vi "edit_waveform.vi"(8 "error in":errorcluster, 9 "units/sec (ms=1000)":dbl=1000.0, 10 "Clock Rate":dbl=1000000.0 min=0.0, 11 "Channels Control":string[][](table)=[["Hex 3D MOT b0", "1", "0", "", "", "", "", "", "", "", "", "", "", "", "", "", "", "", "", ""], ["Hex 3D MOT b0", "1", "0", "", "", "", "", "", "", "", "", "", "", "", "", "", "", "", "", ""], ["repumper bit0", "1", "0", "", "", "", "", "", "", "", "", "", "", "", "", "", "", "", "", ""], ["Trap Array beam switch", "1", "0", "", "", "", "", "", "", "", "", "", "", "", "", "", "", "", "", ""], ["2D MOT switch", "1", "0", "", "", "", "", "", "", "", "", "", "", "", "", "", "", "", "", ""], ["Hamamatsu CCD trigger", "1", "0", "", "", "", "", "", "", "", "", "", "", "", "", "", "", "", "", ""], ["Luca CCD trigger", "1", "0", "", "", "", "", "", "", "", "", "", "", "", "", "", "", "", "", ""], ["broken", "", "", "", "", "", "", "", "", "", "", "", "", "", "", "", "", "", "", ""], ["repumper bit1", "1", "0", "", "", "", "", "", "", "", "", "", "", "", "", "", "", "", "", ""], ["blow away", "1", "0", "", "", "", "", "", "", "", "", "", "", "", "", "", "", "", "", ""], ["trap shutter", "1", "0", "", "", "", "", "", "", "", "", "", "", "", "", "", "", "", "", ""], ["1038 switch", "1", "0", "", "", "", "", "", "", "", "", "", "", "", "", "", "", "", "", ""], ["", "", "", "", "", "", "", "", "", "", "", "", "", "", "", "", "", "", "", ""], ["", "", "", "", "", "", "", "", "", "", "", "", "", "", "", "", "", "", "", ""], ["", "", "", "", "", "", "", "", "", "", "", "", "", "", "", "", "", "", "", ""], ["", "", "", "", "", "", "", "", "", "", "", "", "", "", "", "", "", "", "", ""], ["", "", "", "", "", "", "", "", "", "", "", "", "", "", "", "", "", "", "", ""], ["", "", "", "", "", "", "", "", "", "", "", "", "", "", "", "", "", "", "", ""], ["", "", "", "", "", "", "", "", "", "", "", "", "", "", "", "", "", "", "", ""], ["", "", "", "", "", "", "", "", "", "", "", "", "", "", "", "", "", "", "", ""], ["", "", "", "", "", "", "", "", "", "", "", "", "", "", "", "", "", "", "", ""], ["", "", "", "", "", "", "", "", "", "", "", "", "", "", "", "", "", "", "", ""], ["", "", "", "", "", "", "", "", "", "", "", "", "", "", "", "", "", "", "", ""], ["", "", "", "", "", "", "", "", "", "", "", "", "", "", "", "", "", "", "", ""], ["", "", "", "", "", "", "", "", "", "", "", "", "", "", "", "", "", "", "", ""], ["", "", "", "", "", "", "", "", "", "", "", "", "", "", "", "", "", "", "", ""], ["", "", "", "", "", "", "", "", "", "", "", "", "", "", "", "", "", "", "", ""], ["", "", "", "", "", "", "", "", "", "", "", "", "", "", "", "", "", "", "", ""], ["", "", "", "", "", "", "", "", "", "", "", "", "", "", "", "", "", "", "", ""], ["", "", "", "", "", "", "", "", "", "", "", "", "", "", "", "", "", "", "", ""], ["", "", "", "", "", "", "", "", "", "", "", "", "", "", "", "", "", "", "", ""]]) -> (0 "error out":errorcluster, 3 "Channels out":string[][](table)=[["Hex 3D MOT b0", "1", "0", "", "", "", "", "", "", "", "", "", "", "", "", "", "", "", "", ""], ["Hex 3D MOT b0", "1", "0", "", "", "", "", "", "", "", "", "", "", "", "", "", "", "", "", ""], ["repumper bit0", "1", "0", "", "", "", "", "", "", "", "", "", "", "", "", "", "", "", "", ""], ["Trap Array beam switch", "1", "0", "", "", "", "", "", "", "", "", "", "", "", "", "", "", "", "", ""], ["2D MOT switch", "1", "0", "", "", "", "", "", "", "", "", "", "", "", "", "", "", "", "", ""], ["Hamamatsu CCD trigger", "1", "0", "", "", "", "", "", "", "", "", "", "", "", "", "", "", "", "", ""], ["Luca CCD trigger", "1", "0", "", "", "", "", "", "", "", "", "", "", "", "", "", "", "", "", ""], ["broken", "", "", "", "", "", "", "", "", "", "", "", "", "", "", "", "", "", "", ""], ["repumper bit1", "1", "0", "", "", "", "", "", "", "", "", "", "", "", "", "", "", "", "", ""], ["blow away", "1", "0", "", "", "", "", "", "", "", "", "", "", "", "", "", "", "", "", ""], ["trap shutter", "1", "0", "", "", "", "", "", "", "", "", "", "", "", "", "", "", "", "", ""], ["1038 switch", "1", "0", "", "", "", "", "", "", "", "", "", "", "", "", "", "", "", "", ""], ["", "", "", "", "", "", "", "", "", "", "", "", "", "", "", "", "", "", "", ""], ["", "", "", "", "", "", "", "", "", "", "", "", "", "", "", "", "", "", "", ""], ["", "", "", "", "", "", "", "", "", "", "", "", "", "", "", "", "", "", "", ""], ["", "", "", "", "", "", "", "", "", "", "", "", "", "", "", "", "", "", "", ""], ["", "", "", "", "", "", "", "", "", "", "", "", "", "", "", "", "", "", "", ""], ["", "", "", "", "", "", "", "", "", "", "", "", "", "", "", "", "", "", "", ""], ["", "", "", "", "", "", "", "", "", "", "", "", "", "", "", "", "", "", "", ""], ["", "", "", "", "", "", "", "", "", "", "", "", "", "", "", "", "", "", "", ""], ["", "", "", "", "", "", "", "", "", "", "", "", "", "", "", "", "", "", "", ""], ["", "", "", "", "", "", "", "", "", "", "", "", "", "", "", "", "", "", "", ""], ["", "", "", "", "", "", "", "", "", "", "", "", "", "", "", "", "", "", "", ""], ["", "", "", "", "", "", "", "", "", "", "", "", "", "", "", "", "", "", "", ""], ["", "", "", "", "", "", "", "", "", "", "", "", "", "", "", "", "", "", "", ""], ["", "", "", "", "", "", "", "", "", "", "", "", "", "", "", "", "", "", "", ""], ["", "", "", "", "", "", "", "", "", "", "", "", "", "", "", "", "", "", "", ""], ["", "", "", "", "", "", "", "", "", "", "", "", "", "", "", "", "", "", "", ""], ["", "", "", "", "", "", "", "", "", "", "", "", "", "", "", "", "", "", "", ""], ["", "", "", "", "", "", "", "", "", "", "", "", "", "", "", "", "", "", "", ""], ["", "", "", "", "", "", "", "", "", "", "", "", "", "", "", "", "", "", "", ""]])   [LabVIEW 2013]
doc: "This vi can be used to read a Timing Sequence Control from a file, edit it, and save it to a file.\n\nTo load a file:\nSelect Load. Select or type the path. Execute.\n\nTo save a file:\nEdit the file. Select Save. Select or type the path. Execute."
uses:
  <vilib>/Utility/file.llb/Read From Spreadsheet File (string).vi
  <vilib>/Utility/file.llb/Write To Spreadsheet File (string).vi
panel:
  in  "Variables (Control)":string[][](table)=[["inital period (ms)", "i", "1000", "1000", "1"], ["Overall period (ms)", "t", "5000", "5000", "1"], ["counter rest (ms)", "r", "23", "23", "1"], ["counter pulse (ms)", "c", "2", "2", "1"]] caption="(Inner loop at top)"
  in  "Simulate":bool
  out "output waveform":digitaldata={"transitions"=[0, 75000, 1070000, 1075000, 1080000, 1100000, 1150000, 3005000, 3100000, 3150000, 3200000, 3270000, 3470000, 4999999], "data"=[[0, 0, 0, 0, 0, 0, 1, 0], [1, 0, 0, 0, 0, 0, 1, 0], [1, 0, 0, 1, 1, 0, 1, 0], [0, 0, 0, 1, 1, 0, 1, 0], [0, 1, 0, 1, 1, 0, 1, 0], [0, 0, 1, 1, 1, 0, 1, 1], [0, 0, 1, 1, 1, 0, 1, 0], [0, 0, 1, 1, 1, 0, 1, 0], [0, 0, 0, 1, 1, 0, 1, 0], [0, 0, 0, 1, 1, 0, 1, 1], [0, 0, 0, 1, 1, 0, 1, 0], [0, 0, 0, 0, 0, 0, 1, 0], [0, 0, 0, 0, 0, 0, 1, 0], [0, 0, 0, 0, 0, 0, 1, 0]]}
  out "Digital Waveform Graph":digitaldata(graph)={"transitions"=[0, 75000, 1070000, 1075000, 1080000, 1100000, 1150000, 3005000, 3100000, 3150000, 3200000, 3270000, 3470000, 4999999], "data"=[[0, 0, 0, 0, 0, 0, 1, 0], [1, 0, 0, 0, 0, 0, 1, 0], [1, 0, 0, 1, 1, 0, 1, 0], [0, 0, 0, 1, 1, 0, 1, 0], [0, 1, 0, 1, 1, 0, 1, 0], [0, 0, 1, 1, 1, 0, 1, 1], [0, 0, 1, 1, 1, 0, 1, 0], [0, 0, 1, 1, 1, 0, 1, 0], [0, 0, 0, 1, 1, 0, 1, 0], [0, 0, 0, 1, 1, 0, 1, 1], [0, 0, 0, 1, 1, 0, 1, 0], [0, 0, 0, 0, 0, 0, 1, 0], [0, 0, 0, 0, 0, 0, 1, 0], [0, 0, 0, 0, 0, 0, 1, 0]]}
  in  "Load Waveform from File":bool
  in  "Save Waveform to File":bool
  in  "Exit":bool
  in  "Timing Sequence Control (ms)":string[][](table)=[["Hex 3D MOT DDS bit0", "1", "0", "20.6", "10", "20", "100", "20", "", "", "", "", "", "", "", "", "", "", "", "", "", "", "", "", ""], ["Hex 3D MOT DDS bit1", "1", "0", "20", ".6", "10", "120", "20", "", "", "", "", "", "", "", "", "", "", "", "", "", "", "", "", ""], ["repumper bit0", "1", "0", "29.6", "51", "1000", "", "", "", "", "", "", "", "", "", "", "", "", "", "", "", "", "", "", ""], ["Trap array beam switch", "1", "0", "5", "20", "1000", "", "", "", "", "", "", "", "", "", "", "", "", "", "", "", "", "", "", ""], ["2D MOT switch", "1", "0", "20", "780", "1080", "", "", "", "", "", "", "", "", "", "", "", "", "", "", "", "", "", "", ""], ["Hamamatsu CCD Trigger", "1", "0", "80.6", "10", "", "", "", "", "", "", "", "", "", "", "", "", "", "", "", "", "", "", "", ""], ["Luca CCD trigger", "1", "0", "", "", "", "", "", "", "", "", "", "", "", "", "", "", "", "", "", "", "", "", "", ""], ["broken", "1", "0", "", "", "", "", "", "", "", "", "", "", "", "", "", "", "", "", "", "", "", "", "", ""], ["repumper bit1", "1", "0", "", "", "", "", "", "", "", "", "", "", "", "", "", "", "", "", "", "", "", "", "", ""], ["blow away", "1", "0", "", "", "", "", "", "", "", "", "", "", "", "", "", "", "", "", "", "", "", "", "", ""], ["trap shutter", "1", "0", "", "", "", "", "", "", "", "", "", "", "", "", "", "", "", "", "", "", "", "", "", ""], ["", "1", "0", "", "", "", "", "", "", "", "", "", "", "", "", "", "", "", "", "", "", "", "", "", ""], ["", "1", "0", "", "", "", "", "", "", "", "", "", "", "", "", "", "", "", "", "", "", "", "", "", ""], ["", "1", "0", "", "", "", "", "", "", "", "", "", "", "", "", "", "", "", "", "", "", "", "", "", ""], ["", "1", "0", "", "", "", "", "", "", "", "", "", "", "", "", "", "", "", "", "", "", "", "", "", ""], ["", "1", "0", "", "", "", "", "", "", "", "", "", "", "", "", "", "", "", "", "", "", "", "", "", ""], ["", "1", "0", "", "", "", "", "", "", "", "", "", "", "", "", "", "", "", "", "", "", "", "", "", ""], ["", "1", "0", "", "", "", "", "", "", "", "", "", "", "", "", "", "", "", "", "", "", "", "", "", ""], ["", "1", "0", "", "", "", "", "", "", "", "", "", "", "", "", "", "", "", "", "", "", "", "", "", ""], ["", "1", "0", "", "", "", "", "", "", "", "", "", "", "", "", "", "", "", "", "", "", "", "", "", ""], ["", "1", "0", "", "", "", "", "", "", "", "", "", "", "", "", "", "", "", "", "", "", "", "", "", ""], ["", "1", "0", "", "", "", "", "", "", "", "", "", "", "", "", "", "", "", "", "", "", "", "", "", ""], ["", "1", "0", "", "", "", "", "", "", "", "", "", "", "", "", "", "", "", "", "", "", "", "", "", ""], ["", "", "", "", "", "", "", "", "", "", "", "", "", "", "", "", "", "", "", "", "", "", "", "", ""], ["", "", "", "", "", "", "", "", "", "", "", "", "", "", "", "", "", "", "", "", "", "", "", "", ""], ["", "", "", "", "", "", "", "", "", "", "", "", "", "", "", "", "", "", "", "", "", "", "", "", ""], ["", "", "", "", "", "", "", "", "", "", "", "", "", "", "", "", "", "", "", "", "", "", "", "", ""], ["", "", "", "", "", "", "", "", "", "", "", "", "", "", "", "", "", "", "", "", "", "", "", "", ""], ["Hex 2D MOT on=0/off=1", "1", "0", "", "", "", "", "", "", "", "", "", "", "", "", "", "", "", "", "", "", "", "", "", ""], ["Hex 3D MOT DDS bit0", "1", "0", "", "", "", "", "", "", "", "", "", "", "", "", "", "", "", "", "", "", "", "", "", ""], ["Hex 3D MOT DDS bit1", "1", "0", "", "", "", "", "", "", "", "", "", "", "", "", "", "", "", "", "", "", "", "", "", ""], ["Hex Luca trigger", "1", "0", "", "", "", "", "", "", "", "", "", "", "", "", "", "", "", "", "", "", "", "", "", ""]]
  # "Waveform Simulation"
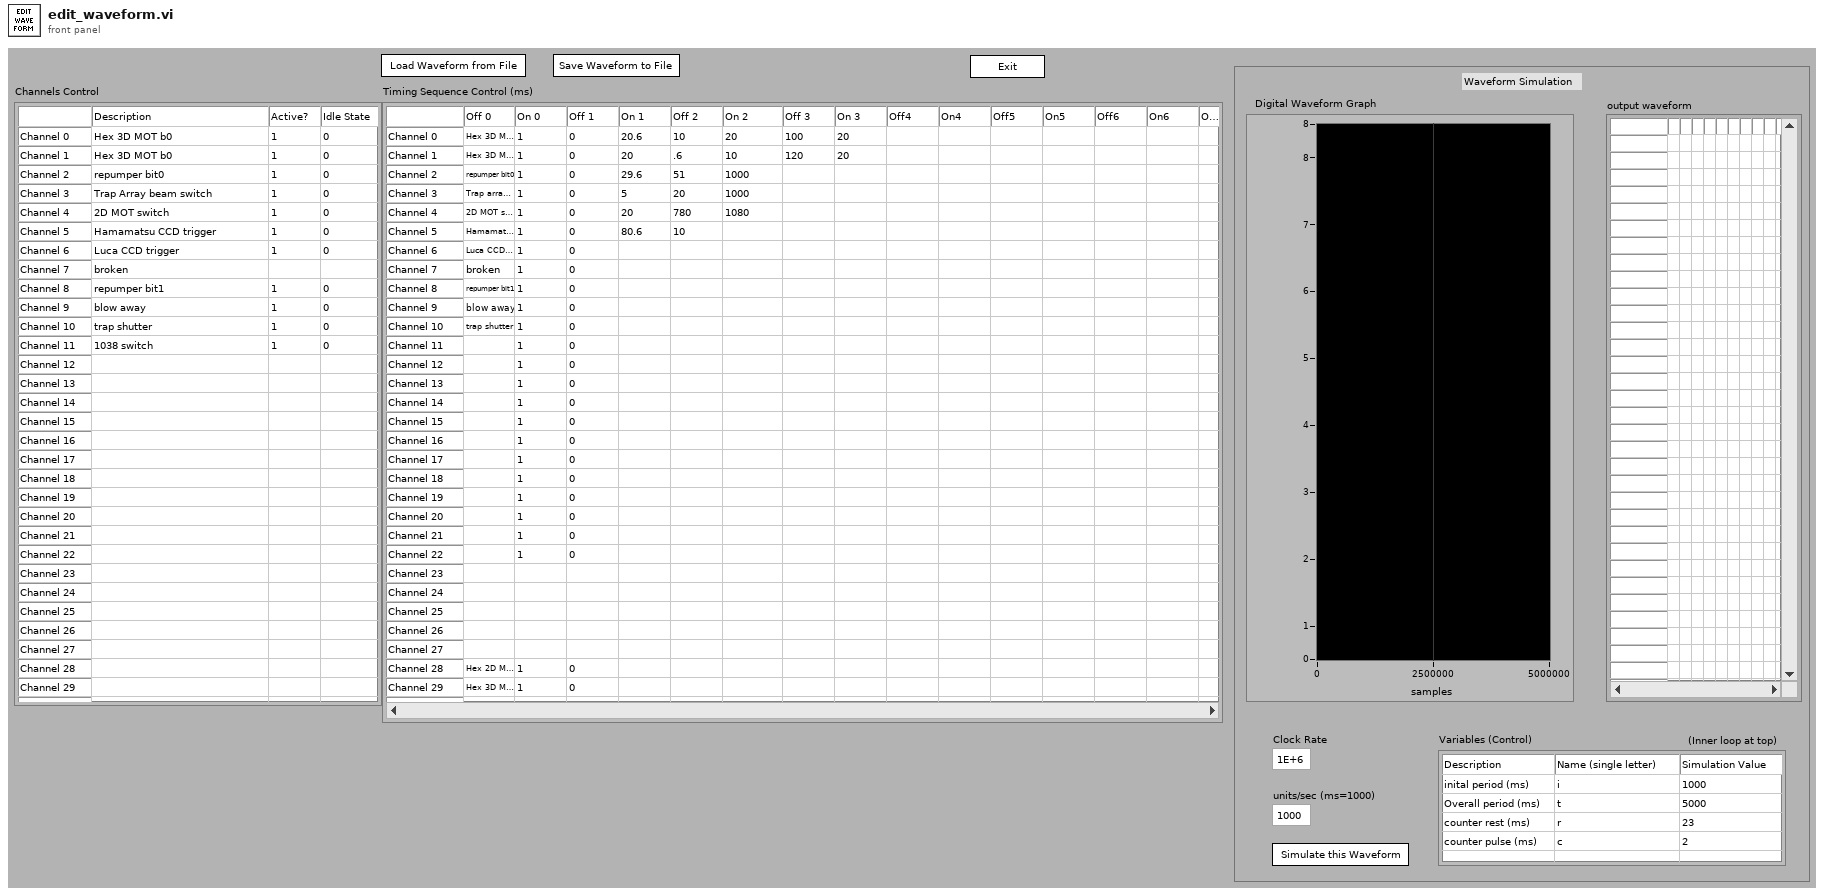
[diagram p1: front panel]
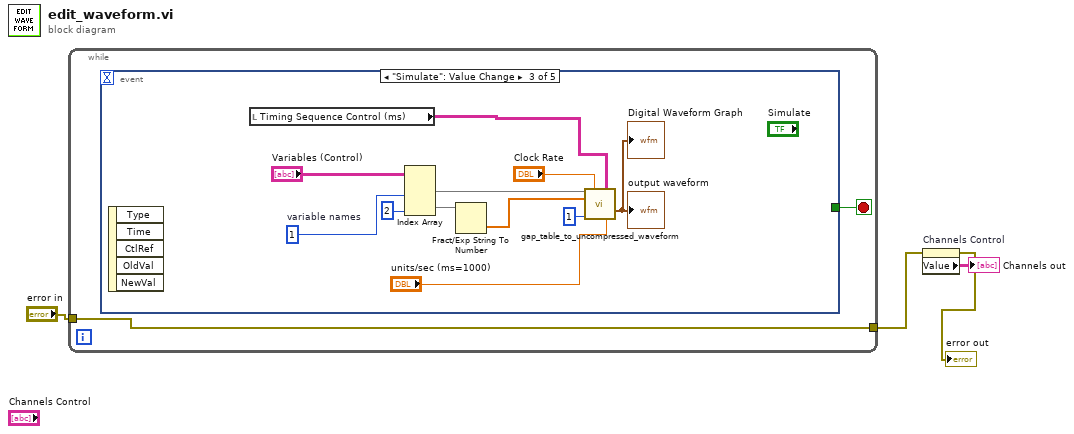
[diagram p0: block diagram]
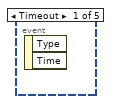
[diagram p2: hidden frame]
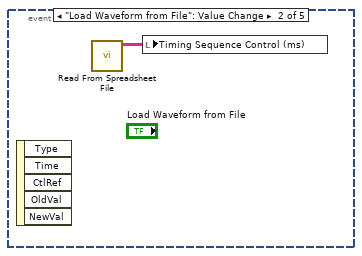
[diagram p3: hidden frame]
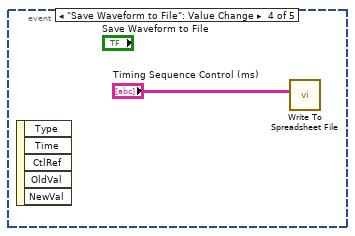
[diagram p4: hidden frame]
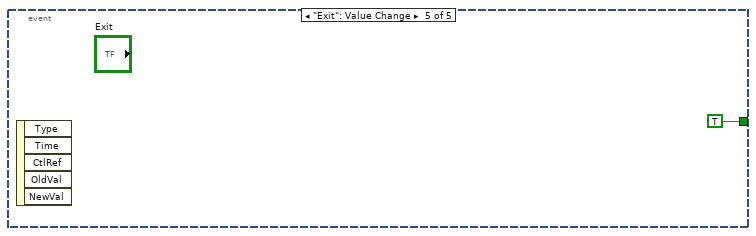
[diagram p5: hidden frame]
diagram:
  n1 = while {
    tunnel: [w5] -> w4
    tunnel: "error in" -> [w5]
    stop <- w6 stop-if-true
    n2 = event shown="[2] \"Simulate\": Value Change" {
      selector: _ -> [_ _ _ _ _]
      dyn-events: _ -> [_ _ _ _ _]
      timeout: _ -> [_ _ _ _ _]
      tunnel: [_ _ _ _ TRUE] -> w6
      event Timeout {
        n3 = event-data() -> ()  [unwired: 1 in, 2 out]
      }
      event "Load Waveform from File": Value Change {
        n4 = event-data() -> ()  [unwired: 1 in, 5 out]
        n5 = call-poly <vilib>:"Read From Spreadsheet File.vi"() -> ("all rows"=w7:string[][])  [unwired: 7 in, 4 out]
        n6 = local write "Timing Sequence Control (ms)"(w7) -> ()
      }
      event "Simulate": Value Change {
        w16 = 1  # variable names
        n7 = event-data() -> ()  [unwired: 1 in, 5 out]
        n8 = local read "Timing Sequence Control (ms)"() -> (w9:string[][])
        n9 = Index Array(array="Variables (Control)", index (col) #1=w16, index (col) #2=2 ("index (col)")) -> (element #1=w15:string[], element #2=w13:string[])  [unwired: 2 in]
        n10 = Fract/Exp String To Number(string=w13) -> (number=w12:dbl[])  [unwired: 3 in, 1 out]
        n11 = call "gap_table_to_uncompressed_waveform.vi"("Variable Names"=w15, "Clock Rate"="Clock Rate", "Timing Sequence Control (ms)"=w9, "Current Value Array"=w12, "HSDIO Settings.Hardware alignment quantum\n(in samples)"=u16 1 ("HSDIO Settings.Hardware alignment quantum\n(in samples)"), "units/sec (ms=1000)"="units/sec (ms=1000)") -> ("output waveform"=→"output waveform" →"Digital Waveform Graph":digitaldata)  [unwired: 5 in, 4 out]
      }
      event "Save Waveform to File": Value Change {
        n12 = event-data() -> ()  [unwired: 1 in, 5 out]
        n13 = call-poly <vilib>:"Write To Spreadsheet File.vi"("2D data"="Timing Sequence Control (ms)") -> ()  [unwired: 7 in, 1 out]
      }
      event "Exit": Value Change {
        n14 = event-data() -> ()  [unwired: 1 in, 5 out]
      }
    }
  }
  n15 = property on="Channels Control" class="Tbl (strict)"(error in=w4) -> (error out=→"error out":errorcluster, "Value"=→"Channels out":string[][])  [unwired: 1 in, 1 out]
